vi "TCP Status Check.vi"(0 "listener ID in":refnum<k5>, 5 "Clients":refnum<k5>[](array[refnum])) -> (6 "Clients":refnum<k5>[](array[refnum]), 8 "send data":bool, 15 "no error":errorcluster)   [LabVIEW 2020, in "TCP Server.lvlib"]
uses:
  TCP Server.lvlib
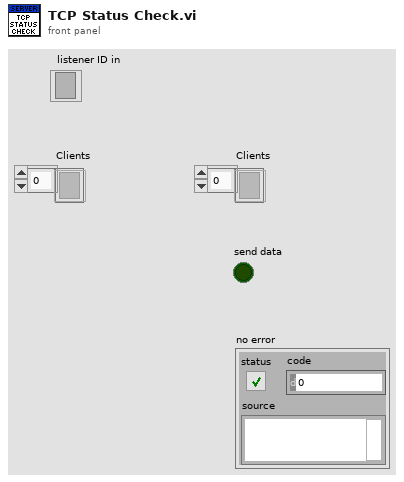
[diagram p1: front panel]
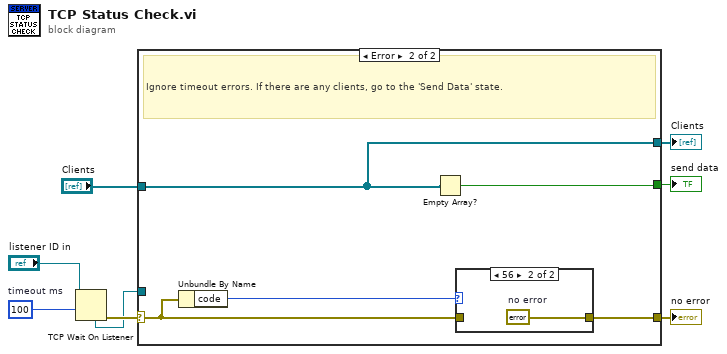
[diagram p0: block diagram]
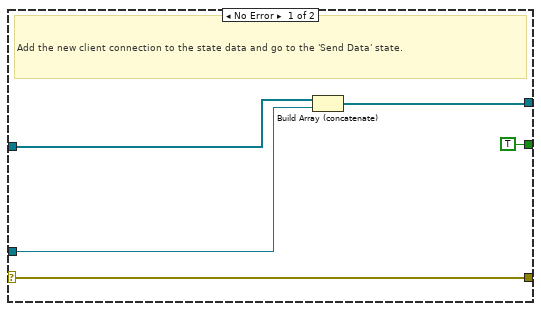
[diagram p2: hidden frame]
diagram:
  w8 = 100  # timeout ms
  n1 = TCP Wait On Listener(9:w8, 11:"listener ID in") -> (0:w7:errorcluster, 4:w1:refnum<k5>)  [unwired: 1 in, 4 out]
  n2 = case shown="Error" w7 {
    selector: w7 -> [w12 w18]
    tunnel: w1 -> [w13 _]
    tunnel: [w12 w16] -> w2
    tunnel: "Clients" -> [w11 w14]
    tunnel: [TRUE ("empty?") w15] -> w4
    tunnel: [w10 w14] -> w3
    frame No Error {
      # "Add the new client connection to the state data and go to the 'Send Data' state."
      n3 = Build Array (concatenate)(w11, w13) -> (w10:refnum<k5>[])
    }
    frame Error {
      # "Ignore timeout errors. If there are any clients, go to the 'Send Data' state."
      n4 = Unbundle By Name(w18) -> ("code"=w17:i32)
      n5 = Empty Array?(array=w14) -> (empty?=w15:bool)
      n6 = case shown="56" w17 {
        tunnel: w18 -> [w19 _]
        tunnel: [w19 w20] -> w16
        frame Default {
        }
        frame 56 {
          w20 = errorcluster {"status"=FALSE, "code"=0, "source"=""}  # no error
        }
      }
    }
  }
  "send data" <- w4
  "Clients" <- w3
  "no error" <- w2
